vi "Node - Reader.vi"(8 "error in (no error)":errorcluster, 9 "Reading Segment":T1, 10 "PXImc Reading Session In":refnum<k21>, 11 "Master Table Ref In":refnum<data-value>) -> (0 "error out":errorcluster)   [LabVIEW 2016, in "PXImc Custom Device Engine.lvlib" / "PXImc Router.lvlib"]
uses:
  PXImc Router.lvlib
  Controls/Table Index-Size.ctl
  Router/Router - Globals.vi
  <vilib>/pximc/Acquire Read Region (DBL).vi
  <resource>/objmgr/pximc.rc
  <vilib>/pximc/nipximc.lvlib
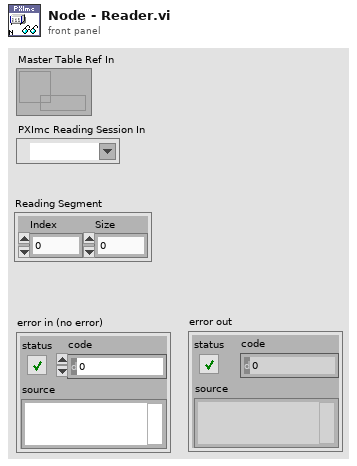
[diagram p1: front panel]
types:
  T1 = typedef "PXImc Custom Device Engine.lvlib/PXImc Router.lvlib/Table Index-Size.ctl" = cluster{"Index":u32, "Size":u32}
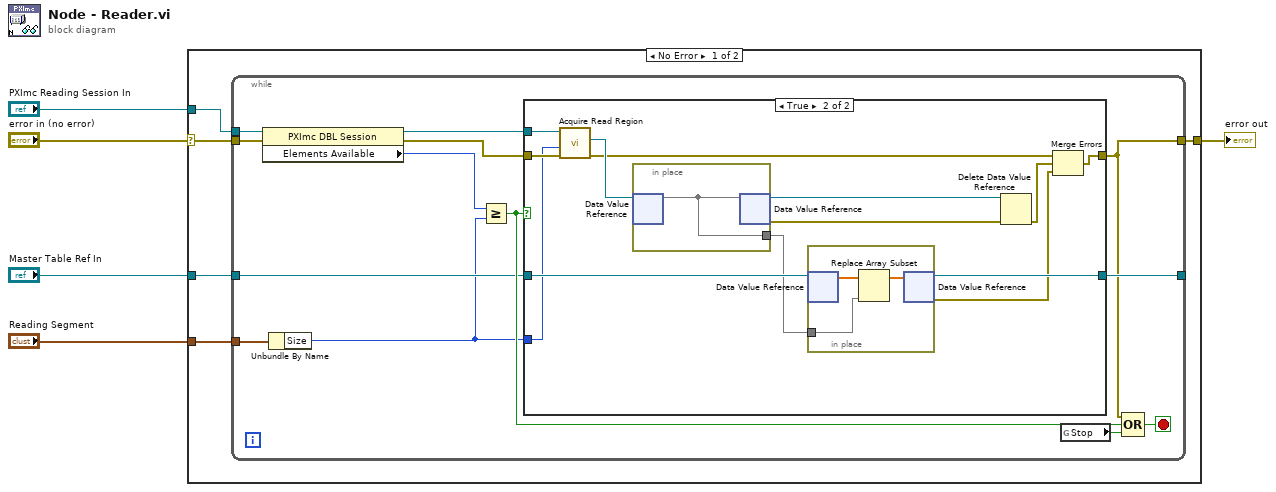
[diagram p0: block diagram]
diagram:
  n1 = case shown="No Error" "error in (no error)" {
    selector: "error in (no error)" -> [w8 w43]
    tunnel: "PXImc Reading Session In" -> [w10 _]
    tunnel: "Master Table Ref In" -> [w9 _]
    tunnel: [w7 w43] -> w4
    tunnel: "Reading Segment" -> [w6 _]
    frame No Error {
      n2 = while {
        tunnel: w10 -> [w23]
        tunnel: w8 -> [w20]
        tunnel: [w13] -> w7
        tunnel: [w18] -> _
        tunnel: w9 -> [w15]
        tunnel: w6 -> [w12]
        stop <- w16 stop-if-true
        n3 = property class="PXImc DBL Session"(reference=w23, error in=w20) -> (reference out=w21:refnum<k21>, error out=w19:errorcluster, "Elements Available"=w22:u64)
        n4 = Unbundle By Name(w12) -> ("Size"=w11:u32)
        n5 = Greater Or Equal?(x=w22, y=w11) -> (x >= y?=w17:bool)
        n6 = case shown="True" w17 {
          tunnel: w19 -> [w25 w37]
          tunnel: [w25 w31] -> w13
          tunnel: w21 -> [_ w36]
          tunnel: [w24 w29] -> w18
          tunnel: w11 -> [_ w27]
          tunnel: w15 -> [w24 w30]
          frame False {
          }
          frame True {
            n7 = call-poly <vilib>:"Acquire Read Region.vi"("error in (no error)"=w37, "number of elements"=w27, "session in"=w36) -> ("error out"=w32:errorcluster, "read region reference"=w38:refnum<data-value>)  [unwired: 5 in, 2 out]
            n8 = in-place {
              in-place-border: [w42] -> w26
              n9 = in-place-dvr #1(w38) -> (w42:dbl[])  [unwired: 1 out]
              n10 = in-place-dvr #1(w42) -> (w35:refnum<data-value>, w34:errorcluster)
            }
            n11 = in-place {
              in-place-border: w26 -> [w39]
              n12 = in-place-dvr #2(w30) -> (w41:dbl[])  [unwired: 1 out]
              n13 = Replace Array Subset(array=w41, new element=w39) -> (w40:dbl[])  [unwired: 1 in]
              n14 = in-place-dvr #2(w40) -> (w29:refnum<data-value>, w28:errorcluster)
            }
            n15 = Delete Data Value Reference(data value reference=w35, error in=w34) -> (error out=w33:errorcluster)  [unwired: 1 out]
            n16 = Merge Errors(w32, w33, w28) -> (w31:errorcluster)
          }
        }
        n17 = global read "Router - Globals.vi" "Stop"() -> (w14:bool)
        n18 = Compound Arithmetic op=OR(w13, w17, w14) -> (w16:bool)
      }
    }
    frame Error {
    }
  }
  "error out" <- w4
